vi "sintriangleprofile.vi"() -> ()   [LabVIEW 2023]
uses:
  <vilib>/Analysis/NI_AALBase.lvlib
panel:
  in  "SineFrequency":dbl
  in  "SineAmplitude":dbl
  out "Added Waveform":dbl[](graph)
  out "Waveform2":dbl[](graph)
  out "Waveform1":dbl[](graph)
  in  "TriangleAmplitude":dbl
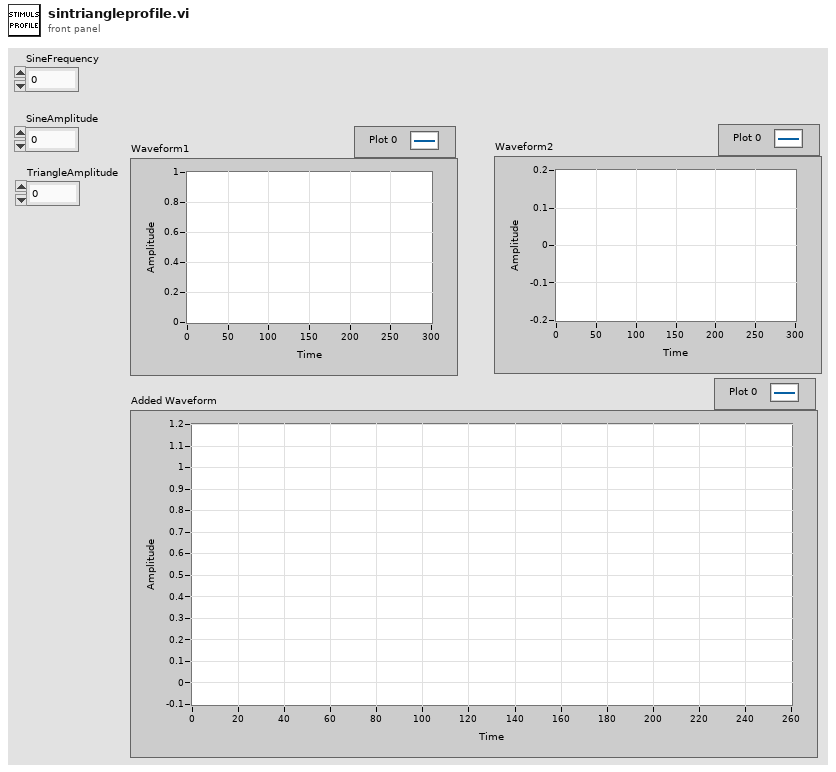
[diagram p1: front panel]
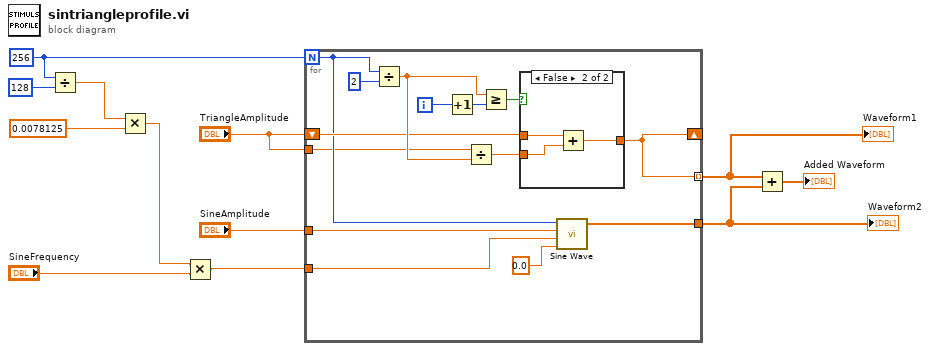
[diagram p0: block diagram]
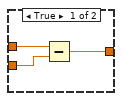
[diagram p2: hidden frame]
diagram:
  w6 = 256
  n1 = Divide(x=w6, y=128) -> (x/y=w4:dbl)
  n2 = Multiply(x=w4, y=0.0078125 ("frequency")) -> (x*y=w2:dbl)
  n3 = Multiply(x=w2, y="SineFrequency") -> (x*y=w1:dbl)
  n4 = for {
    N: w6 -> [w16]
    shift-right: [w19] -> _
    shift-left: "TriangleAmplitude" -> [w21]
    tunnel: [w19] -> w12 mode=indexing
    tunnel: [w17] -> w11
    tunnel: "SineAmplitude" -> [w18]
    tunnel: w1 -> [w13]
    tunnel: "TriangleAmplitude" -> [w14]
    i -> [w25]
    n5 = Divide(x=w16, y=2) -> (x/y=w22:dbl)
    n6 = Increment(x=w25) -> (x+1=w24:i32)
    n7 = Divide(x=w14, y=w22) -> (x/y=w20:dbl)
    n8 = Greater Or Equal?(x=w22, y=w24) -> (x >= y?=w23:bool)
    n9 = case shown="False" w23 {
      tunnel: w21 -> [w29 w32]
      tunnel: [w28 w31] -> w19
      tunnel: w20 -> [w27 w30]
      frame True {
        n10 = Subtract(x=w29, y=w27) -> (x-y=w28:dbl)
      }
      frame False {
        n11 = Add(x=w32, y=w30) -> (x+y=w31:dbl)
      }
    }
    n12 = call <vilib>:"Sine Wave.vi"("samples"=w16, "amplitude"=w18, "frequency"=w13, "phase in"=0.0) -> ("sine wave"=w17:dbl[])  [unwired: 1 in, 2 out]
  }
  "Waveform2" <- w11
  "Waveform1" <- w12
  n13 = Add(x=w12, y=w11) -> (x+y=→"Added Waveform":dbl[])
